vi "RedisplayCurve.vi"(11 "UiDefinition 3":T1) -> ()   [LabVIEW 2020]
uses:
  UIReferences.ctl
  D:/LabviewDXFViewer/LabviewDXFViewer/bin/Release/LabviewDXFViewer.exe
  LabviewDXFViewer/bin/Release/LabviewDXFViewer.exe
  <vilib>/Utility/file.llb/Read Delimited Spreadsheet (DBL).vi
panel:
  out "error out":errorcluster
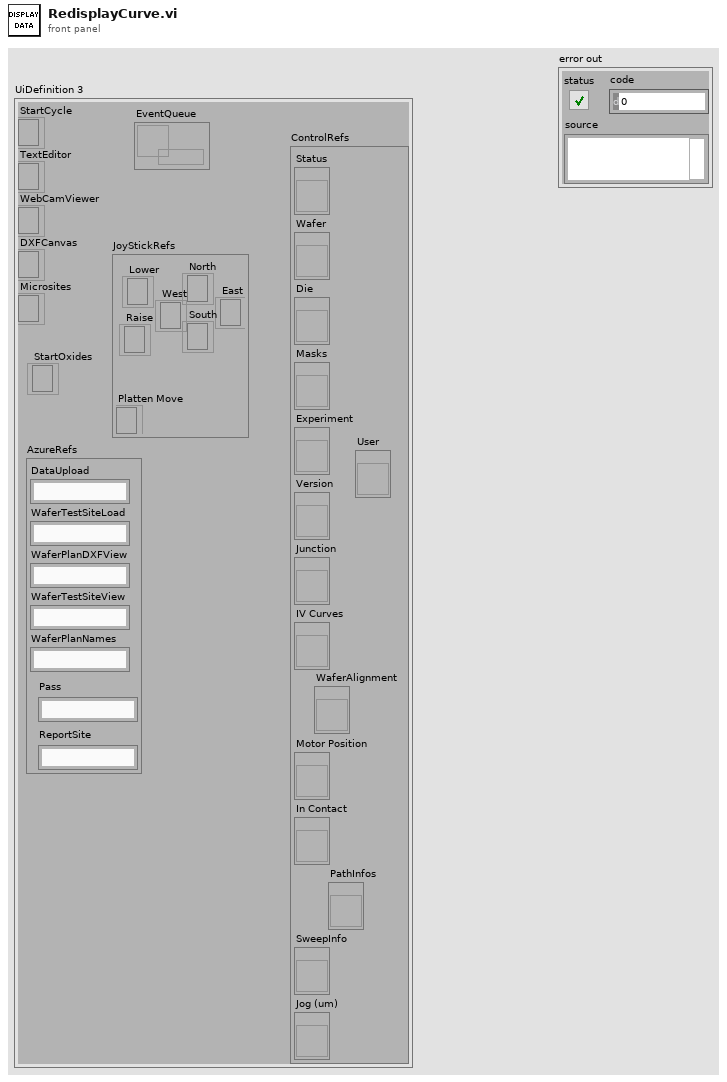
[diagram p1: front panel]
types:
  T1 = typedef "UIReferences.ctl" = cluster{"StartCycle":refnum<k24>, "TextEditor":refnum<k24>, "WebCamViewer":refnum<k24>, "DXFCanvas":refnum<k24>, "Microsites":refnum<k24>, "JoyStickRefs":cluster{"North":refnum<k24>, "Lower":refnum<k24>, "Raise":refnum<k24>, "Platten Move":refnum<k24>, "West":refnum<k24>, "East":refnum<k24>, "South":refnum<k24>}, "AzureRefs":cluster{"DataUpload":string, "WaferTestSiteLoad":string, "WaferPlanDXFView":string, "WaferTestSiteView":string, "WaferPlanNames":string, "Pass":string, "ReportSite":string}, "ControlRefs":cluster{"Status":refnum<vi>, "Wafer":refnum<vi>, "Die":refnum<vi>, "Masks":refnum<vi>, "Experiment":refnum<vi>, "Version":refnum<vi>, "Junction":refnum<vi>, "IV Curves":refnum<vi>, "Motor Position":refnum<vi>, "In Contact":refnum<vi>, "SweepInfo":refnum<vi>, "Jog (um)":refnum<vi>, "PathInfos":refnum<vi>, "User":refnum<vi>, "WaferAlignment":refnum<vi>}, "EventQueue":refnum<queue>, "StartOxides":refnum<k24>}
  T2 = cluster{"Die":string, "Wafer":string, "Path":path, "url":string, "Experiment":string, "Version":string, "user":string}
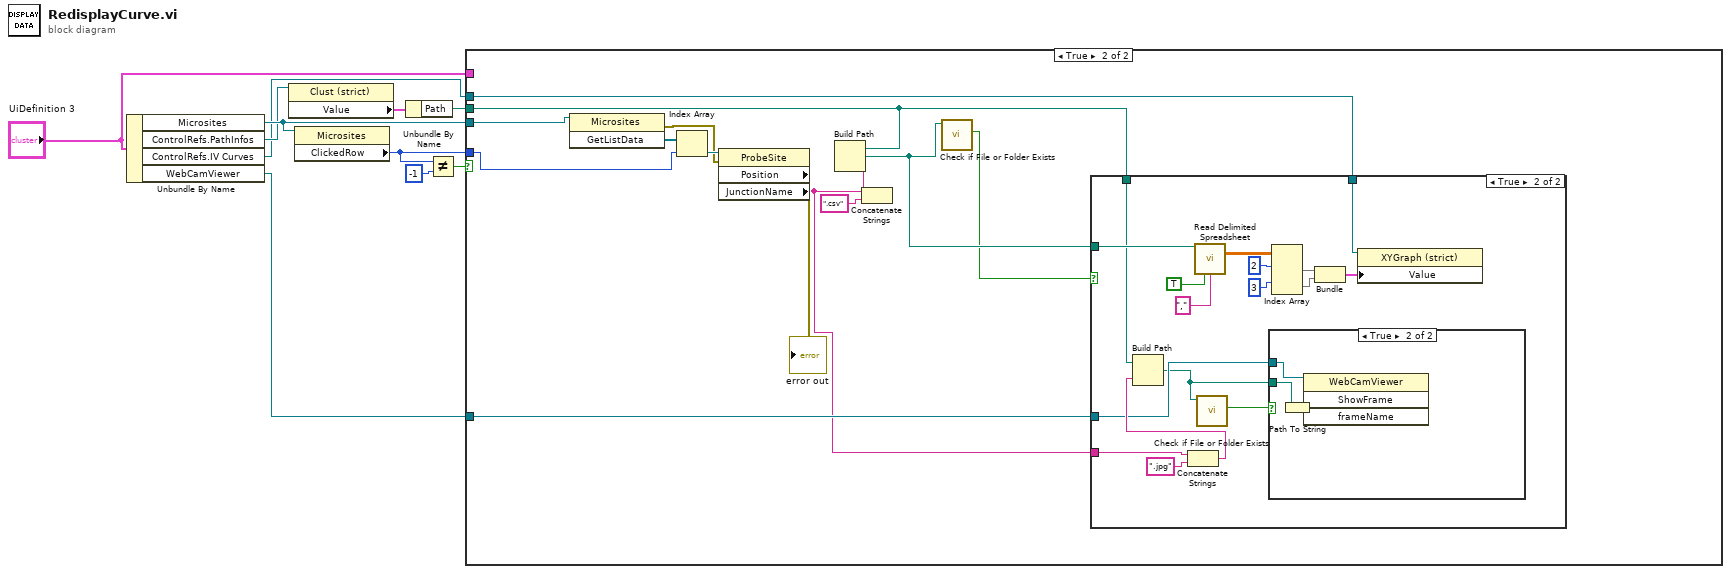
[diagram p0: block diagram]
diagram:
  n1 = Unbundle By Name("UiDefinition 3") -> ("Microsites"=w6:refnum<k24>, "ControlRefs.PathInfos"=w5:refnum<vi>, "ControlRefs.IV Curves"=w2:refnum<vi>, "WebCamViewer"=w1:refnum<k24>)
  n2 = property class="Clust (strict)"(reference=w5) -> ("Value"=w4:T2)  [unwired: 1 in, 2 out]
  n3 = property class="Microsites"(reference=w6) -> ("ClickedRow"=w9:i32)  [unwired: 1 in, 2 out]
  n4 = Unbundle By Name(w4) -> ("Path"=w3:path)
  n5 = Not Equal?(x=w9, y=-1) -> (x != y?=w8:bool)
  n6 = case shown="True" w8 {
    tunnel: w9 -> [_ w21]
    tunnel: "UiDefinition 3" -> [_ _]
    tunnel: w6 -> [_ w22]
    tunnel: w3 -> [_ w12]
    tunnel: w2 -> [_ w18]
    tunnel: w1 -> [_ w13]
    frame False {
    }
    frame True {
      n7 = invoke class="Microsites" method="GetListData"(reference=w22) -> (error out=w15:errorcluster, "GetListData"=w24:refnum<k24>[])  [unwired: 2 in, 1 out]
      n8 = Index Array(array=w24, index=w21) -> (element=w23:refnum<k24>)
      n9 = property class="ProbeSite" props=["Position", "JunctionName"](reference=w23, error in=w15) -> (error out=→"error out":errorcluster, "JunctionName"=w11:string)  [unwired: 2 out]
      n10 = Concatenate Strings(w11, ".csv" ("string")) -> (w19:string)
      n11 = Build Path(base path=w12, name or relative path=w19) -> (appended path=w17:path)
      n12 = call <vilib>:"Check if File or Folder Exists.vi"("path"=w17) -> ("file or folder exists?"=w16:bool)  [unwired: 8 in, 2 out]
      n13 = case shown="True" w16 {
        tunnel: w18 -> [_ w41]
        tunnel: w17 -> [_ w34]
        tunnel: w13 -> [_ w26]
        tunnel: w12 -> [_ w29]
        tunnel: w11 -> [_ w28]
        frame False {
        }
        frame True {
          n14 = Concatenate Strings(w28, ".jpg" ("string")) -> (w30:string)
          n15 = Build Path(base path=w29, name or relative path=w30) -> (appended path=w25:path)
          n16 = call-poly <vilib>:"Read Delimited Spreadsheet.vi"("file path (dialog if empty)"=w34, "transpose? (F)"=TRUE, "delimiter (\\t)"="," ("delimiter (\\t)")) -> ("all rows"=w39:dbl[][])  [unwired: 7 in, 5 out]
          n17 = call <vilib>:"Check if File or Folder Exists.vi"("path"=w25) -> ("file or folder exists?"=w27:bool)  [unwired: 8 in, 2 out]
          n18 = case shown="True" w27 {
            tunnel: w26 -> [_ w44]
            tunnel: w25 -> [_ w43]
            frame False {
            }
            frame True {
              n19 = Path To String(path=w43) -> (string=w42:string)
              n20 = invoke class="WebCamViewer" method="ShowFrame"(reference=w44, "frameName"=w42) -> ()  [unwired: 2 in, 4 out]
            }
          }
          n21 = Index Array(array=w39, index (row) #1=2 ("index (row)"), index (row) #2=3 ("index (row)")) -> (element #1=w36:dbl[], element #2=w35:dbl[])  [unwired: 2 in]
          n22 = Bundle("all rows"=w36, "all rows"=w35) -> (w40:cluster{"all rows":dbl[], "all rows":dbl[]})  [unwired: 1 in]
          n23 = property class="XYGraph (strict)"(reference=w41, "Value"=w40) -> ()  [unwired: 1 in, 2 out]
        }
      }
    }
  }
